vi "showOCRResultwithBB.vi"(6 "error in":errorcluster, 7 "Array":T2[](array[typedef]), 8 "chars":u8[](array[numeric]), 9 "Image in":T1) -> (0 "error out":errorcluster, 3 "Image out":T1)   [LabVIEW 2025, in "adsOCR.lvlib" / "ocr.lvclass"]
uses:
  ocr.lvclass
  TextDecRecResult2L.ctl
  <vilib>/vision/Image Controls.llb/IMAQ Image.ctl
  ocr.lvclass/ocr.ctl
panel:
  in  "Image In":T1(plugin-control)
  out "Image":T1(plugin-control)
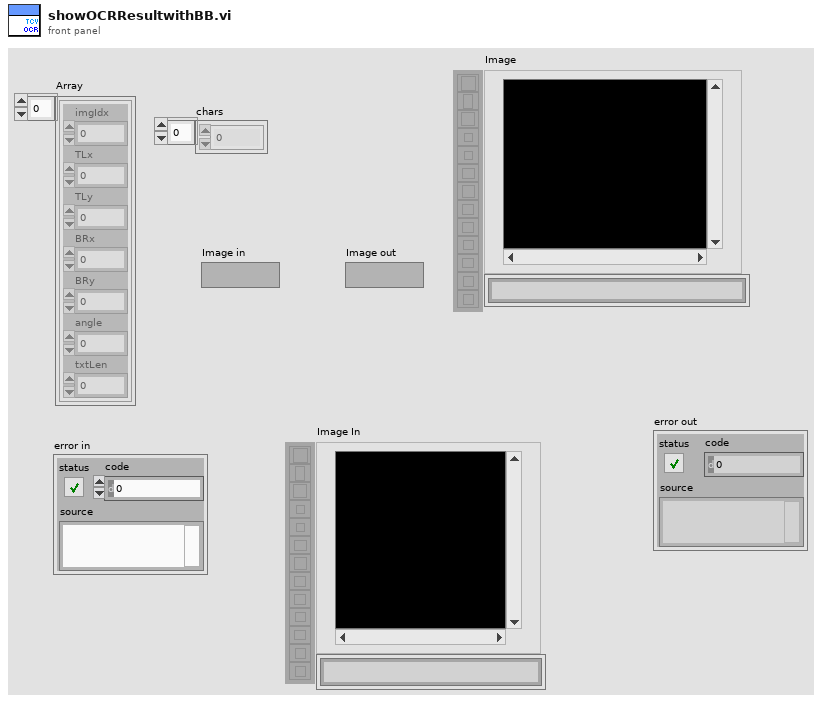
[diagram p1: front panel]
types:
  T1 = typedef "IMAQ Image.ctl" = refnum<image>
  T2 = typedef "adsOCR.lvlib/ocr.lvclass/TextDecRecResult2L.ctl" = cluster{"imgIdx":i32, "TLx":i32, "TLy":i32, "BRx":i32, "BRy":i32, "angle":sgl, "txtLen":i32}
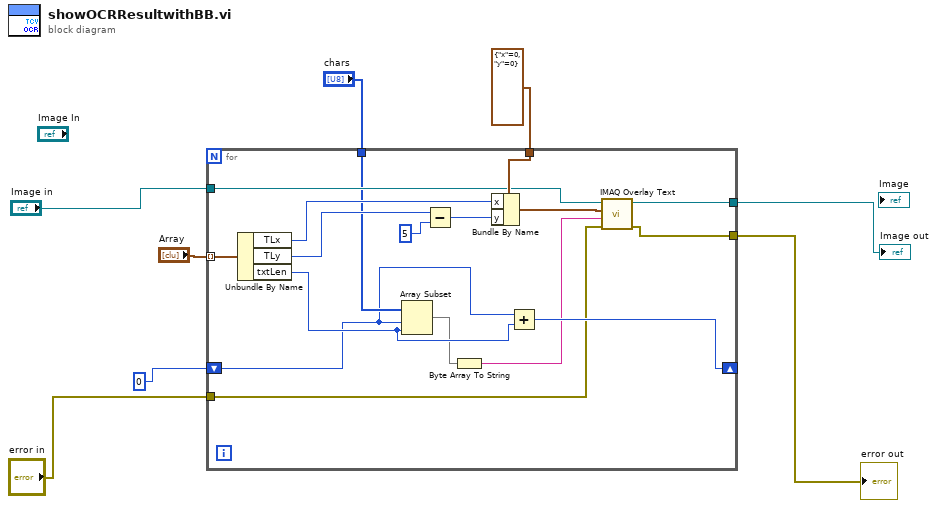
[diagram p0: block diagram]
diagram:
  n1 = for {
    tunnel: "Array" -> [w25] mode=indexing
    tunnel: cluster{"x":i32, "y":i32} {"x"=0, "y"=0} -> [w22]
    tunnel: "Image in" -> [w18]
    shift-right: [w16] -> _
    shift-left: 0 -> [w14]
    tunnel: "chars" -> [w17]
    tunnel: [w11] -> w1
    tunnel: "error in" -> [w10]
    tunnel: [w9] -> w3
    n2 = Unbundle By Name(w25) -> ("TLx"=w21:i32, "TLy"=w24:i32, "txtLen"=w15:i32)
    n3 = Array Subset(array=w17, index=w14, length=w15) -> (w13:u8[])
    n4 = Subtract(x=w24, y=5) -> (x-y=w20:i32)
    n5 = Byte Array To String(unsigned byte array=w13) -> (string=w12:string)
    n6 = Bundle By Name(cluster=w22, "x"=w21, "y"=w20) -> (w19:cluster{"x":i32, "y":i32})
    n7 = Add(x=w14, y=w15) -> (x+y=w16:i32)
    n8 = call "IMAQ Overlay Text"("error in (no error)"=w10, "String"=w12, "Origin"=w19, "Image"=w18) -> ("error out"=w9:errorcluster, "Image Out"=w11:T1)  [unwired: 6 in]
  }
  "error out" <- w3
  "Image out" <- w1
